vi "Time To Milliseconds.vi"(2 "Input Time [s]":dbl) -> (6 "Output Time [ms]":dbl)   [LabVIEW 2014]
doc: "Convert time in seconds to milleseconds."
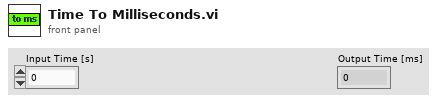
[diagram p1: front panel]
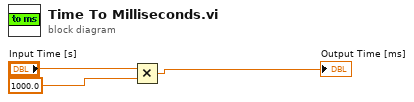
[diagram p0: block diagram]
diagram:
  n1 = Multiply(x="Input Time [s]", y=1000.0) -> (x*y=→"Output Time [ms]":dbl)
